vi "New.vi"(8 "error in (no error)":errorcluster, 11 "reference in":refnum<class "MES_Base.lvclass">) -> (0 "error out":errorcluster, 3 "reference out":refnum<class "MES_Base.lvclass">)   [LabVIEW 2022 SP3, in "MES_Base.lvlib" / "MES_Base.lvclass"]
uses:
  MES_Base.lvclass
  ObjectAttributes.ctl
  Config.ctl
  MES_Base.lvclass/MES_Base.ctl
  Components/ViPER.lvlibp/ViPER.lvclass
panel:
  in  "Data":T1
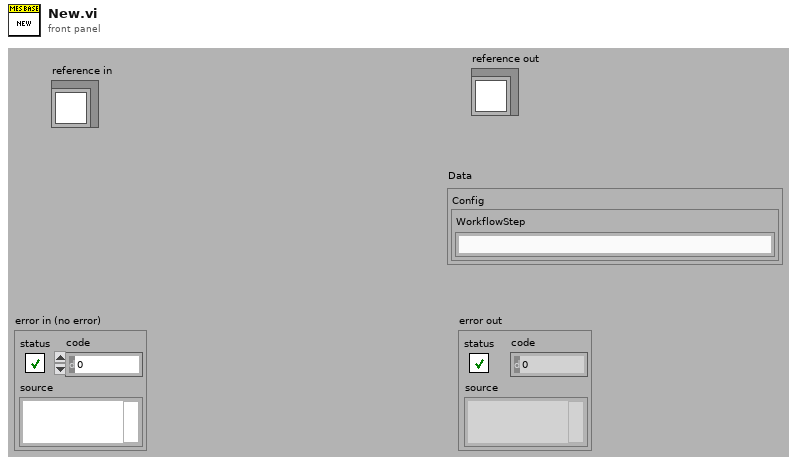
[diagram p1: front panel]
types:
  T1 = typedef "MES_Base.lvlib/MES_Base.lvclass/ObjectAttributes.ctl" = cluster{"Config":T2}
  T2 = typedef "MES_Base.lvlib/MES_Base.lvclass/Config.ctl" = cluster{"WorkflowStep":string}
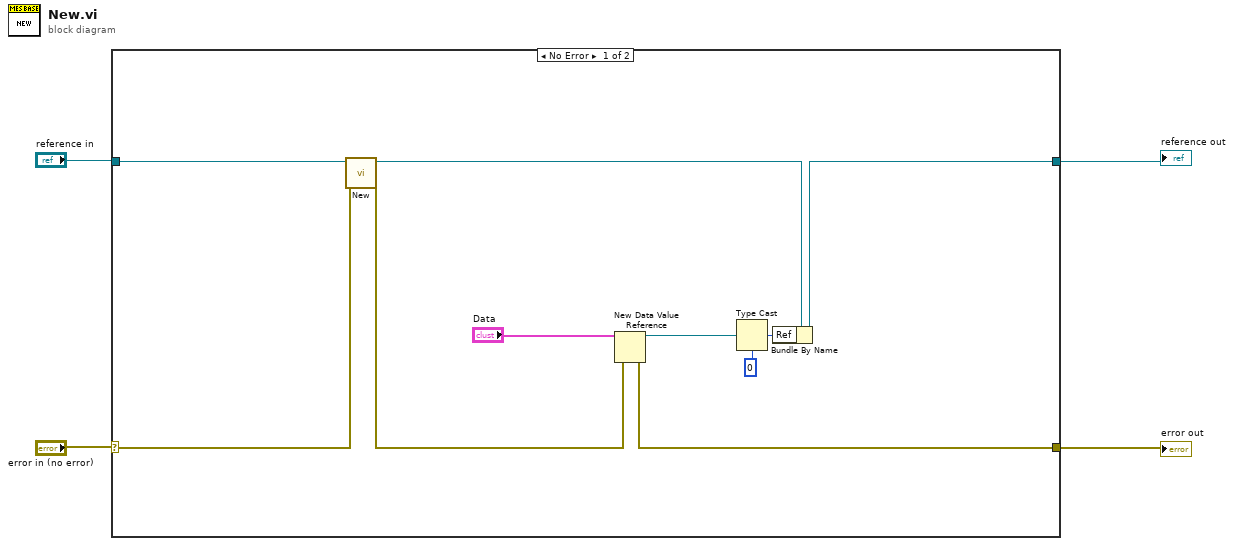
[diagram p0: block diagram]
diagram:
  n1 = case shown="No Error" "error in (no error)" {
    selector: "error in (no error)" -> [w6 w16]
    tunnel: [w7 w16] -> w2
    tunnel: "reference in" -> [w14 w15]
    tunnel: [w13 w15] -> w1
    frame No Error {
      n2 = call-parent "New.vi"("error in (no error)"=w6, "reference in"=w14) -> ("error out"=w5:errorcluster, "reference out"=w12:refnum<class "MES_Base.lvclass">)  [unwired: 8 in]
      n3 = New Data Value Reference(data value="Data", error in=w5) -> (data value reference=w10:refnum<data-value>, error out=w7:errorcluster)
      n4 = Type Cast(type=u32 0 ("DataRef"), x=w10) -> (*(type *) &x=w9:u32)
      n5 = Bundle By Name(cluster=w12, "Ref"=w9) -> (w13:refnum<class "MES_Base.lvclass">)
    }
    frame Error {
    }
  }
  "error out" <- w2
  "reference out" <- w1
